vi "Read Min Depth Message.vi"(8 "error in (no error)":errorcluster, 11 "AIP Set Min Depth Message in":refnum<class "AIP Set Min Depth Message.lvclass">) -> (0 "error out":errorcluster, 2 "Min Depth":u8, 3 "AIP Set Min Depth Message out":refnum<class "AIP Set Min Depth Message.lvclass">)   [LabVIEW 2015, in "RDS Child Messages.lvlib" / "AIP Set Min Depth Message.lvclass"]
uses:
  AIP Set Min Depth Message.lvclass
  AIP Set Min Depth Message.lvclass/AIP Set Min Depth Message.ctl
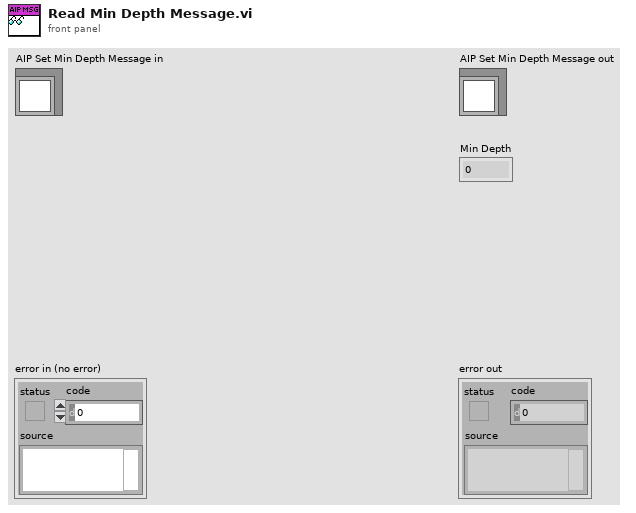
[diagram p1: front panel]
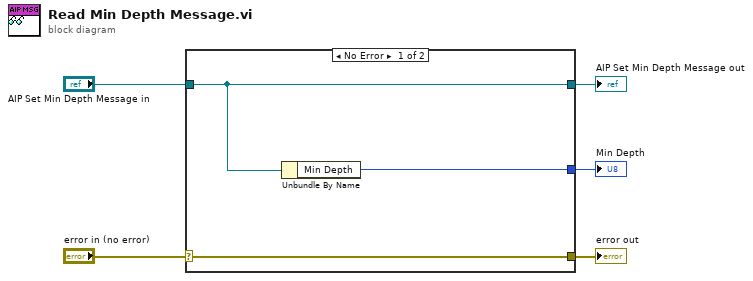
[diagram p0: block diagram]
diagram:
  n1 = case shown="No Error" "error in (no error)" {
    selector: "error in (no error)" -> [w8 w9]
    tunnel: [w8 w9] -> w4
    tunnel: [w7 w10] -> w2
    tunnel: "AIP Set Min Depth Message in" -> [w7 w10]
    tunnel: [w6 _] -> w1
    frame No Error {
      n2 = Unbundle By Name(w7) -> ("Min Depth"=w6:u8)
    }
    frame Error {
    }
  }
  "error out" <- w4
  "AIP Set Min Depth Message out" <- w2
  "Min Depth" <- w1
